vi "Logging Construct.vi"(8 "error in":errorcluster, 11 "identifier":string) -> (0 "error out":errorcluster, 3 "logging execution unit out":refnum<class "Logging Execution Unit.lvclass">)   [LabVIEW 2020, in "AIM ARINC 429 Engine.lvlib" / "Implementation.lvlib" / "Logging Execution Unit.lvclass"]
uses:
  Logging Execution Unit.lvclass
  Custom Device/Hardware Handles.ctl
  Custom Device/Custom Device.lvlib
  Execution Unit/Execution Unit.lvclass
  C:/Git/niveristand-aim-arinc429-custom-device/Source/Custom Device Support/Engine/Implementation/Execution Unit/Execution Unit.lvclass
  C:/Git/niveristand-aim-arinc429-custom-device/Source/Custom Device Support/Engine/Interfaces/Execution Unit/Execution Unit.lvclass
  C:/Git/niveristand-aim-arinc429-custom-device/Source/Custom Device Support/Engine/Implementation/Logging Execution Unit/Logging Execution Unit.lvclass
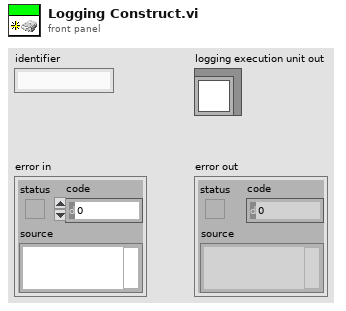
[diagram p1: front panel]
types:
  T1 = typedef "AIM ARINC 429 Engine.lvlib/Custom Device.lvlib/Hardware Handles.ctl" = cluster{"module":u8}
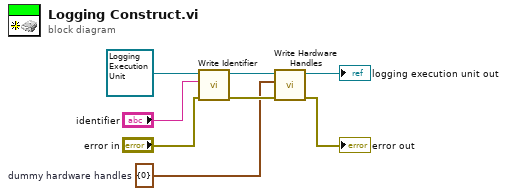
[diagram p0: block diagram]
diagram:
  w1 = T1 {"module"=0}  # dummy hardware handles
  n1 = call "Write Identifier.vi"("error in (no error)"="error in", "identifier"="identifier", "Ballard ARINC-429 Execution Unit in"=refnum<class "Logging Execution Unit.lvclass"> refnum ("Logging Execution Unit out")) -> ("error out"=w5:errorcluster, "Ballard ARINC-429 Execution Unit out"=w6:refnum<class "Logging Execution Unit.lvclass">)  [unwired: 7 in]
  n2 = call "Write Hardware Handles.vi"("error in"=w5, "hardware handles"=w1, "AIM ARINC-429 execution unit in"=w6) -> ("error out"=→"error out":errorcluster, "AIM ARINC-429 execution unit out"=→"logging execution unit out":refnum<class "Logging Execution Unit.lvclass">)  [unwired: 7 in]
